vi "flatten and unflatten test.vi"() -> (0 "serialization error":errorcluster, 3 "pass":bool)   [LabVIEW 2015, in "Tagbus PID Module tests.lvlib"]
uses:
  testing/Tagbus PID Module tests.lvlib
  PID Module configuration.lvclass
  PID Loop.lvclass
  <vilib>/NI/Configuration Framework/serializable configuration/NISE_CEF_serializable configuration.lvclass
panel:
  out "version":string
  out "data":string
  out "output range":cluster{"output high":dbl, "output low":dbl}
  out "PID gains":T1
  out "PID Parameters":T2
  out "ID":string
  in  "error in (no error)":errorcluster
  out "flattened PID Loop":string
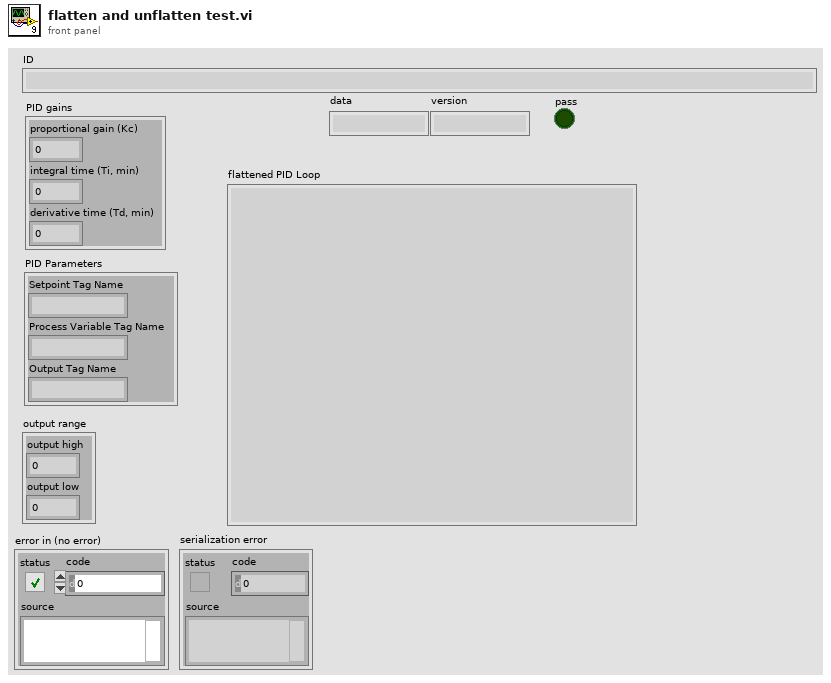
[diagram p1: front panel]
types:
  T1 = cluster{"proportional gain (Kc)":dbl, "integral time (Ti, min)":dbl, "derivative time (Td, min)":dbl}
  T2 = cluster{"Setpoint Tag Name":string, "Process Variable Tag Name":string, "Output Tag Name":string}
  T3 = typedef "PID Parameters.ctl" = cluster{"Setpoint Tag":string, "Process Variable Tag":string, "Output Tag":string}
  T4 = typedef "PID Gains.ctl" = cluster{"proportional gain (Kc)":dbl, "integral time (Ti, min)":dbl, "derivative time (Td, min)":dbl}
  T5 = typedef "PID Range.ctl" = cluster{"output high":dbl, "output low":dbl}
  T6 = typedef "PID Module configuration.lvclass/PID array element.ctl" = cluster{"Loop ID":string, "Tags":cluster{"Setpoint":string, "Process Variable":string, "Output":string}, "Gains":cluster{"P":dbl, "I":dbl, "D":dbl}, "Range":cluster{"High":dbl, "Low":dbl}}
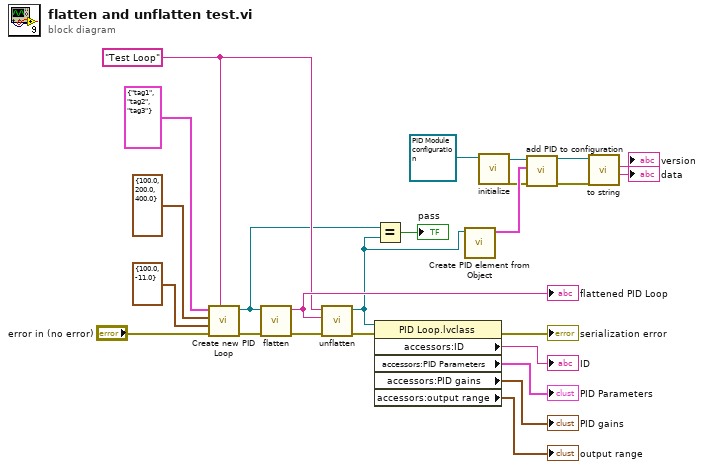
[diagram p0: block diagram]
diagram:
  w18 = "Test Loop" ("ID")
  n1 = call "Create new PID Loop.vi"("ID"=w18, "error in (no error)"="error in (no error)", "output range"=cluster{"output high":dbl, "output low":dbl} {"output high"=100.0, "output low"=-11.0}, "PID gains"=T1 {"proportional gain (Kc)"=100.0, "integral time (Ti, min)"=200.0, "derivative time (Td, min)"=400.0}, "PID Parameters"=T2 {"Setpoint Tag Name"="tag1", "Process Variable Tag Name"="tag2", "Output Tag Name"="tag3"}) -> ("error out"=w25:errorcluster, "PID Loop out"=w11:refnum<class "PID Loop.lvclass">)  [unwired: 5 in]
  n2 = call-dynamic "flatten.vi"("error in (no error)"=w25, "PID Loop in"=w11) -> ("error out"=w20:errorcluster, "flattened PID Loop"=w19:string)  [unwired: 8 in]
  "flattened PID Loop" <- w19
  n3 = call "unflatten.vi"("error in (no error)"=w20, "PID Loop String"=w19, "Identifier"=w18) -> ("error out"=w16:errorcluster, "PID Loop out"=w6:refnum<class "PID Loop.lvclass">)  [unwired: 7 in]
  n4 = Equal?(x=w11, y=w6) -> (x = y?=→"pass":bool)
  n5 = property class="PID Loop.lvclass"(reference=w6, error in=w16) -> (error out=→"serialization error":errorcluster, "accessors:ID"=→"ID":string, "accessors:PID Parameters"=→"PID Parameters":T3, "accessors:PID gains"=→"PID gains":T4, "accessors:output range"=→"output range":T5)  [unwired: 1 out]
  n6 = call "Create PID element from Object.vi"("PID Loop in"=w6) -> ("line"=w5:T6)  [unwired: 10 in]
  n7 = call <vilib>:"initialize.vi"("configuration in"=refnum<class "PID Module configuration.lvclass"> refnum ("Tagbus PID Module configuration in")) -> ("error out"=w4:errorcluster, "configuration out"=w8:refnum<class "PID Module configuration.lvclass">)  [unwired: 8 in, 1 out]
  n8 = call "add PID to configuration.vi"("error in"=w4, "PID Element in"=w5, "Tagbus PID Module configuration in"=w8) -> ("error out"=w3:errorcluster, "Tagbus PID Module configuration out"=w7:refnum<class "PID Module configuration.lvclass">)  [unwired: 7 in]
  n9 = call-dynamic "to string.vi"("error in"=w3, "Tagbus PID Module configuration in"=w7) -> ("data"=→"data":string, "version"=→"version":string)  [unwired: 6 in, 2 out]
